vi "saveUniqueName.vi"(8 "error in (no error)":errorcluster, 10 "Check existence before modifying path":bool=TRUE, 11 "path":path) -> (0 "error out":errorcluster, 3 "unique path":path)   [LabVIEW 2011]
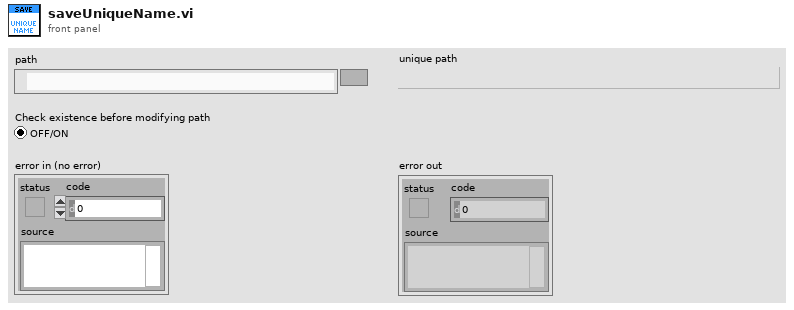
[diagram p1: front panel]
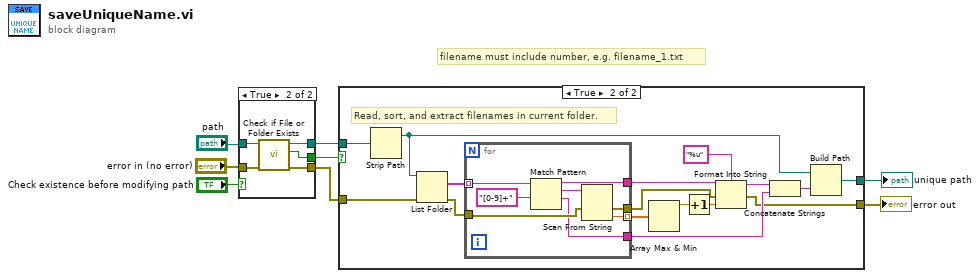
[diagram p0: block diagram]
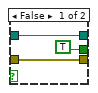
[diagram p2: hidden frame]
diagram:
  # "filename must include number, e.g. filename_1.txt"
  n1 = case shown="True" "Check existence before modifying path" {
    tunnel: "path" -> [w11 w16]
    tunnel: [w11 w15] -> w3
    tunnel: [TRUE ("file or folder exists?") w14] -> w6
    tunnel: "error in (no error)" -> [w9 w13]
    tunnel: [w9 w12] -> w1
    frame False {
    }
    frame True {
      n2 = call <vilib>:"Check if File or Folder Exists.vi"("error in (no error)"=w13, "path"=w16) -> ("error out"=w12:errorcluster, "file or folder exists?"=w14:bool, "dup path"=w15:path)  [unwired: 7 in]
    }
  }
  n3 = case shown="True" w6 {
    tunnel: w3 -> [w18 w33]
    tunnel: [w18 w34] -> w4
    tunnel: [w17 w23] -> w2
    tunnel: w1 -> [w17 w22]
    frame False {
    }
    frame True {
      # "Read, sort, and extract filenames in current folder."
      n4 = Strip Path(path=w33) -> (stripped path=w32:path)  [unwired: 1 out]
      n5 = List Folder(path=w32, error in=w22) -> (filenames=w31:string[], error out=w25:errorcluster)  [unwired: 2 in, 2 out]
      n6 = for {
        tunnel: w31 -> [w42] mode=indexing
        tunnel: [w36] -> w28
        tunnel: [w41] -> w29 mode=indexing
        tunnel: [w39] -> w20
        tunnel: w25 -> [w38]
        tunnel: [w37] -> w24
        n7 = Match Pattern(string=w42, regular expression="[0-9]+") -> (before substring=w36:string, match substring=w35:string, after substring=w37:string)  [unwired: 1 in, 1 out]
        n8 = Scan From String(input string=w35, error in=w38) -> (error out=w39:errorcluster, output 1=w41:dbl)  [unwired: 3 in, 2 out]
      }
      n9 = Array Max & Min(array=w29) -> (max value=w21:dbl)  [unwired: 3 out]
      n10 = Increment(x=w21) -> (x+1=w30:dbl)
      n11 = Format Into String(format string="%u", initial string=w28, error in=w20, w30) -> (resulting string=w27:string, error out=w23:errorcluster)
      n12 = Concatenate Strings(w27, w24) -> (w26:string)
      n13 = Build Path(base path=w32, name or relative path=w26) -> (appended path=w34:path)
    }
  }
  "unique path" <- w4
  "error out" <- w2
